vi "New.vi"(9 "Enums as Strings? (T)":bool=TRUE, 10 "UTC Timestamps? (T)":bool=TRUE, 11 "Pretty Print? (F)":bool) -> (3 "JSON formatter":refnum<class "JSON.lvclass">)   [LabVIEW 2018, in "Logging.lvlib" / "JSON.lvclass"]
uses:
  JSON.lvclass
  JSON.lvclass/JSON.ctl
panel:
  # "Connector Pane"
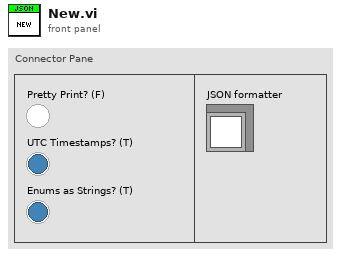
[diagram p1: front panel]
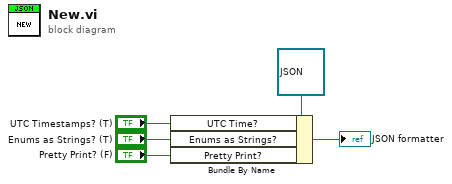
[diagram p0: block diagram]
diagram:
  n1 = Bundle By Name(cluster=refnum<class "JSON.lvclass"> refnum ("JSON formatter"), "UTC Time?"="UTC Timestamps? (T)", "Enums as Strings?"="Enums as Strings? (T)", "Pretty Print?"="Pretty Print? (F)") -> (→"JSON formatter":refnum<class "JSON.lvclass">)
